vi "Get Process from Map.vi"(8 "error in (no error)":errorcluster, 10 "Process Name":string, 11 "Application In":refnum<class "Application.lvclass">) -> (0 "error out":errorcluster, 2 "Process":refnum<class "Process.lvclass">, 3 "Application Out":refnum<class "Application.lvclass">)   [LabVIEW 2020, in "Application.lvclass"]
uses:
  Application.lvclass
  Process/Process.lvclass
  Application.lvclass/Application.ctl
  <vilib>/Utility/error.llb/Error Cluster From Error Code.vi
  <vilib>/ErrorRing/Error Ring.xnode
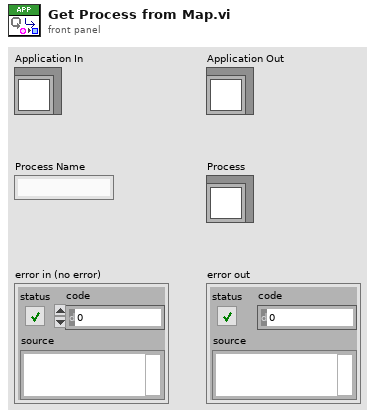
[diagram p1: front panel]
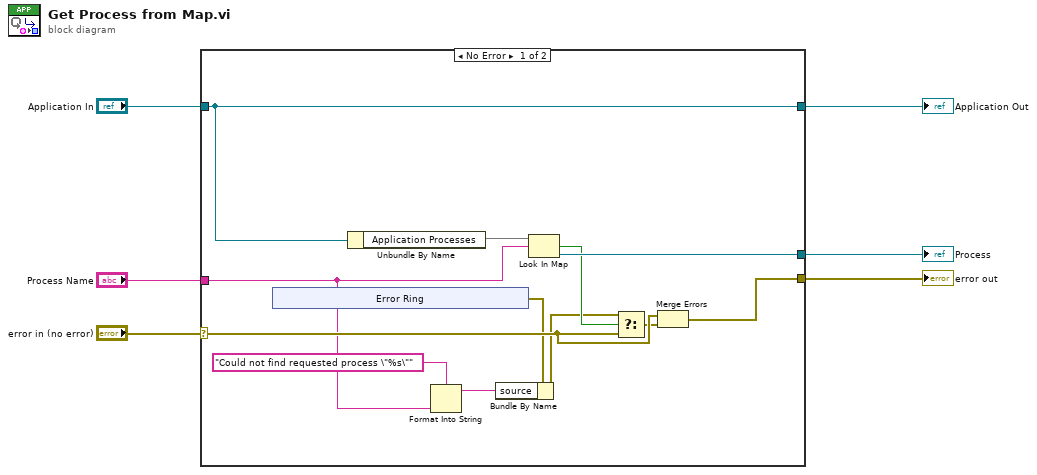
[diagram p0: block diagram]
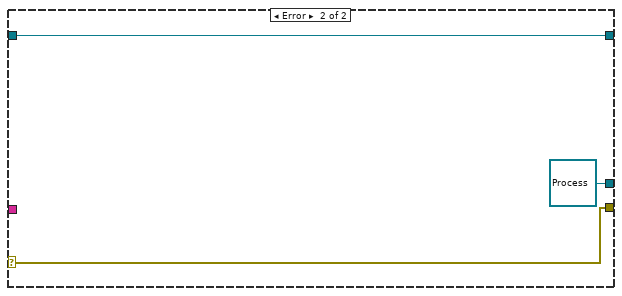
[diagram p2: hidden frame]
diagram:
  n1 = case shown="No Error" "error in (no error)" {
    selector: "error in (no error)" -> [w15 w25]
    tunnel: [w18 refnum<class "Process.lvclass"> refnum ("Process")] -> w6
    tunnel: [w17 w25] -> w5
    tunnel: [w16 w24] -> w4
    tunnel: "Application In" -> [w16 w24]
    tunnel: "Process Name" -> [w8 _]
    frame No Error {
      n2 = xnode "Error Ring"() -> ("error out"=w13:errorcluster)
      n3 = Unbundle By Name(w16) -> ("Application Processes"=w11:map{string, refnum<class "Process.lvclass">})
      n4 = Format Into String(format string="Could not find requested process \"%s\"", w8) -> (resulting string=w7:string)  [unwired: 2 in, 1 out]
      n5 = Bundle By Name(cluster=w13, "source"=w7) -> (w10:errorcluster)
      n6 = Look In Map(map=w11, key=w8) -> (key not found?=w12:bool, value=w18:refnum<class "Process.lvclass">)  [unwired: 1 in]
      n7 = Select(t=w10, s=w12, f=w15) -> (s? t:f=w14:errorcluster)
      n8 = Merge Errors(w15, w14) -> (w17:errorcluster)
    }
    frame Error {
    }
  }
  "Process" <- w6
  "error out" <- w5
  "Application Out" <- w4
